vi "niRFUtil MEAS Validate Complex Waveform.vi"(8 "error in (no error)":errorcluster, 11 "Complex Waveform In":T1 {"y" format="%.2f"; "dx" format="%^.2e"; "x0" format="%^.2e"}) -> (0 "error out":errorcluster, 3 "Complex Waveform Out":T1 {"y" format="%.2f"; "dx" format="%^.2e"; "x0" format="%^.2e"})   [LabVIEW 2015, in "niRFUtil.lvlib"]
uses:
  niRFUtil.lvlib
  Includes/niRFUtil INC Complex Waveform.ctl
  Includes/niRFUtil INC Complex Array.ctl
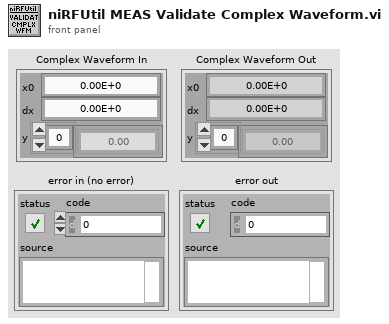
[diagram p1: front panel]
types:
  T1 = typedef "niRFUtil.lvlib/niRFUtil INC Complex Waveform.ctl" = cluster{"x0":dbl, "dx":dbl, "y":T2}
  T2 = typedef "niRFUtil.lvlib/niRFUtil INC Complex Array.ctl" = csg[]
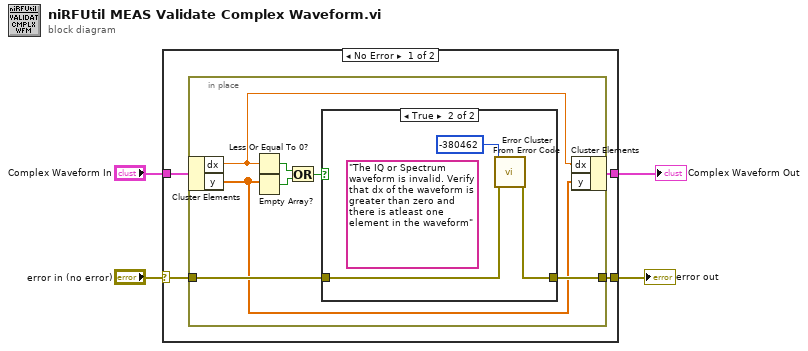
[diagram p0: block diagram]
diagram:
  n1 = case shown="No Error" "error in (no error)" {
    selector: "error in (no error)" -> [w7 w21]
    tunnel: "Complex Waveform In" -> [w6 w20]
    tunnel: [w8 w21] -> w4
    tunnel: [w5 w20] -> w1
    frame No Error {
      n2 = in-place {
        in-place-border: [w12] -> w8
        in-place-border: w7 -> [w11]
        n3 = in-place-cluster #1(w6) -> ("dx"=w10:dbl, "y"=w9:T2)
        n4 = Less Or Equal To 0?(x=w10) -> (x <= 0?=w15:bool)
        n5 = Empty Array?(array=w9) -> (empty?=w14:bool)
        n6 = Or(x=w15, y=w14) -> (x .or. y?=w13:bool)
        n7 = case shown="True" w13 {
          tunnel: w11 -> [w16 w18]
          tunnel: [w16 w17] -> w12
          frame False {
          }
          frame True {
            (unwired) "The IQ or Spectrum waveform is invalid. Verify that dx of the waveform is greater than zero and there is atleast one element in the waveform" ("error message (\"\")")
            n8 = call <vilib>:"Error Cluster From Error Code.vi"("error in (no error)"=w18, "error code (0)"=-380462) -> ("error out"=w17:errorcluster)  [unwired: 7 in]
          }
        }
        n9 = in-place-cluster #1("dx"=w10, "y"=w9) -> (w5:T1)
      }
    }
    frame Error {
    }
  }
  "error out" <- w4
  "Complex Waveform Out" <- w1
